vi "HRM-Stage4-calculate_heartrate.vi"(8 "error in (no error)":errorcluster, 11 "Process data":T1={"Samples size (10)"=10, "Addition signal to remove"=0.0, "Unfiltered wf"={"t0"=timestamp(0 s since 1904-01-01), "dt"=1.0, "Y"=[]}, "Filtered wf"={"t0"=timestamp(0 s since 1904-01-01), "dt"=1.0, "Y"=[]}, "Heart Rate"=0.0, "Peak detect settings"={"Manual?"=FALSE, "Top"=0.0, "Bot"=0.0}, "User Events"={"Signal to remove"=refnum, "Sample size"=refnum, "Filtered wf"=refnum, "Unfiltered wf"=refnum, "Raw wf"=refnum, "Pulse"=refnum, "Stop"=refnum, "Feedback"=refnum, "Run Aqn?"=refnum, "Clear"=refnum, "Peak Det. Set."=refnum}}) -> (0 "error out":errorcluster, 3 "Process data out":T1={"Samples size (10)"=10, "Addition signal to remove"=0.0, "Unfiltered wf"={"t0"=timestamp(0 s since 1904-01-01), "dt"=1.0, "Y"=[]}, "Filtered wf"={"t0"=timestamp(0 s since 1904-01-01), "dt"=1.0, "Y"=[]}, "Heart Rate"=0.0, "Peak detect settings"={"Manual?"=FALSE, "Top"=0.0, "Bot"=0.0}, "User Events"={"Signal to remove"=refnum, "Sample size"=refnum, "Filtered wf"=refnum, "Unfiltered wf"=refnum, "Raw wf"=refnum, "Pulse"=refnum, "Stop"=refnum, "Feedback"=refnum, "Run Aqn?"=refnum, "Clear"=refnum, "Peak Det. Set."=refnum}})   [LabVIEW 2020]
uses:
  HRM-process-loop_cluster.ctl
  HRM-process-peak_detect_setting.ctl
  initclose/HRM-Stage4-User_events.ctl
  <vilib>/measure/matone.llb/Extract Single Tone Information 1 Chan.vi
  <vilib>/measure/NI_MAPro.lvlib
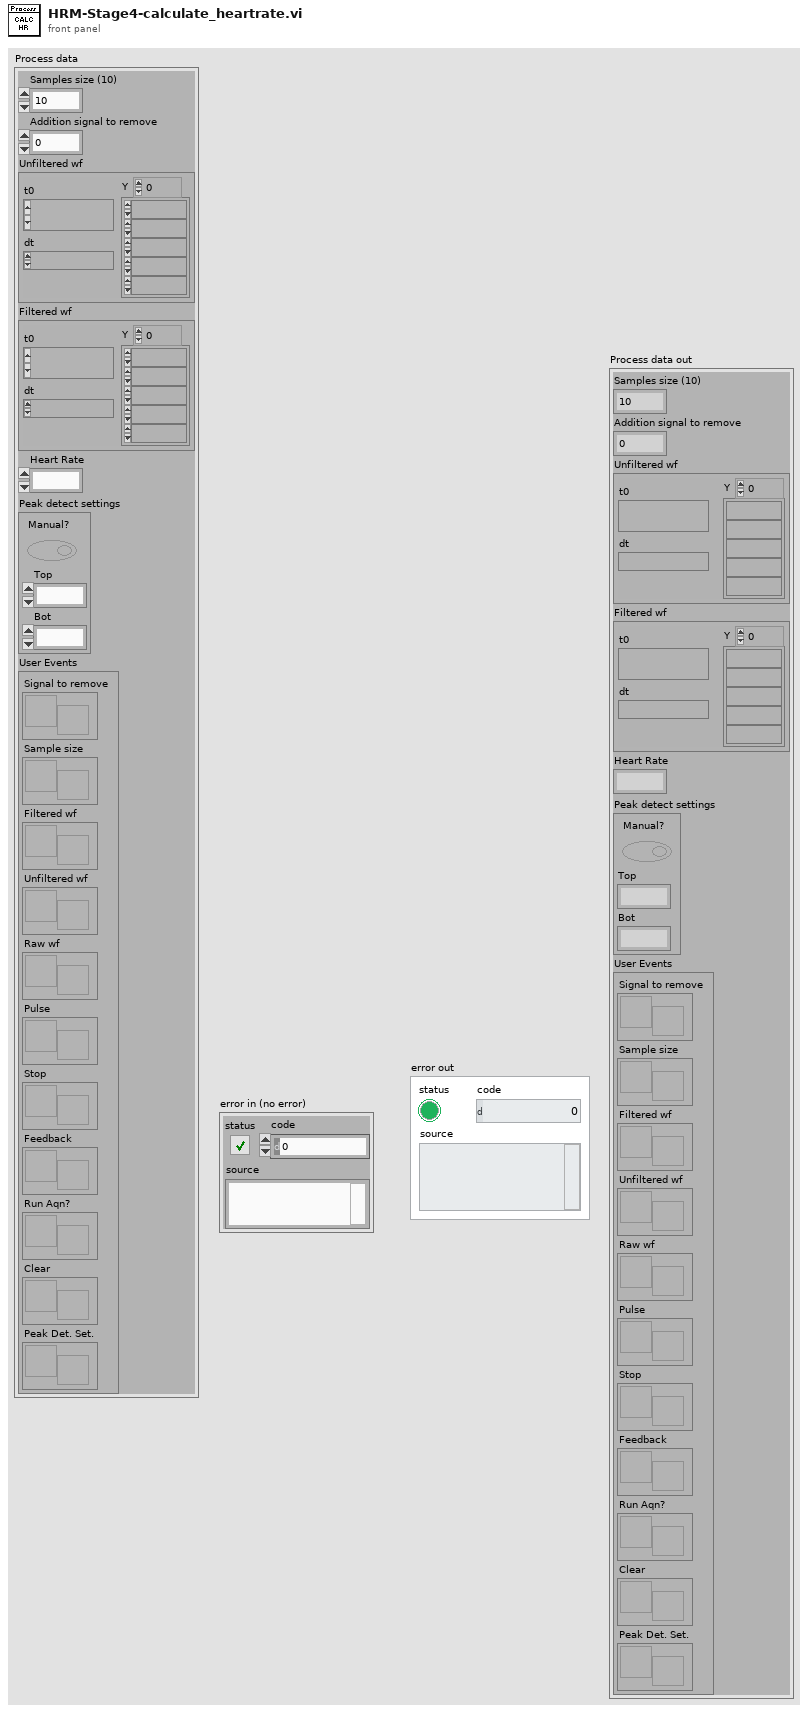
[diagram p1: front panel]
types:
  T1 = typedef "HRM-process-loop_cluster.ctl" = cluster{"Samples size (10)":i32, "Addition signal to remove":dbl, "Unfiltered wf":waveform(dbl), "Filtered wf":waveform(dbl), "Heart Rate":dbl, "Peak detect settings":T2, "User Events":T3}
  T2 = typedef "HRM-process-peak_detect_setting.ctl" = cluster{"Manual?":bool, "Top":dbl, "Bot":dbl}
  T3 = typedef "HRM-Stage4-User_events.ctl" = cluster{"Signal to remove":refnum<user-event>, "Sample size":refnum<user-event>, "Filtered wf":refnum<user-event>, "Unfiltered wf":refnum<user-event>, "Raw wf":refnum<user-event>, "Pulse":refnum<user-event>, "Stop":refnum<user-event>, "Feedback":refnum<user-event>, "Run Aqn?":refnum<user-event>, "Clear":refnum<user-event>, "Peak Det. Set.":refnum<user-event>}
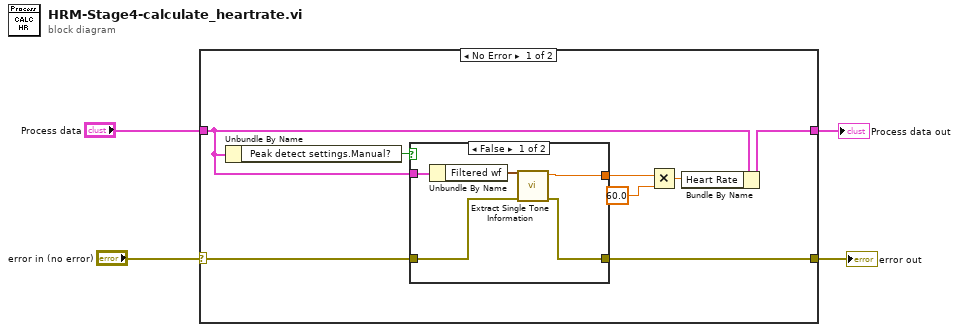
[diagram p0: block diagram]
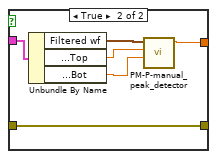
[diagram p2: hidden frame]
diagram:
  n1 = case shown="No Error" "error in (no error)" {
    selector: "error in (no error)" -> [w11 w25]
    tunnel: [w10 w25] -> w3
    tunnel: "Process data" -> [w9 w24]
    tunnel: [w12 w24] -> w1
    frame No Error {
      n2 = Unbundle By Name(w9) -> ("Peak detect settings.Manual?"=w8:bool)
      n3 = case shown="False" w8 {
        tunnel: w11 -> [w17 w19]
        tunnel: [w16 w19] -> w10
        tunnel: w9 -> [w15 w23]
        tunnel: [w13 w18] -> w6
        frame False {
          n4 = Unbundle By Name(w15) -> ("Filtered wf"=w14:waveform(dbl))
          n5 = call-poly <vilib>:"Extract Single Tone Information.vi"("error in (no error)"=w17, "time signal in"=w14) -> ("error out"=w16:errorcluster, "detected frequency"=w13:dbl)  [unwired: 4 in, 4 out]
        }
        frame True {
          n6 = Unbundle By Name(w23) -> ("Filtered wf"=w22:waveform(dbl), "Peak detect settings.Top"=w21:dbl, "Peak detect settings.Bot"=w20:dbl)
          n7 = call "PM-P-manual_peak_detector.vi"("Bot"=w20, "Top"=w21, "waveform in"=w22) -> ("Frequency [Hz]"=w18:dbl)  [unwired: 7 in, 1 out]
        }
      }
      n8 = Multiply(x=w6, y=60.0) -> (x*y=w5:dbl)
      n9 = Bundle By Name(cluster=w9, "Heart Rate"=w5) -> (w12:T1)
    }
    frame Error {
    }
  }
  "Process data out" <- w1
  "error out" <- w3
